vi "Subtract.vi"(7 "LabVIEW Web Service Request":refnum<class "Web Request.lvclass"> caption="LabVIEW Web服务请求", 8 "b":dbl, 11 "a":dbl) -> (2 "value":string, 3 "c":dbl)   [LabVIEW 2014]
uses:
  <vilib>/wsapi/Web Request.lvclass
panel:
  in  "variable name":string(combo) caption="变量名称"
  # "Web服务请求输入接线端用于调用“Web服务”选板的VI。除非不需要访问该选板，否则不要在连线板上删除这个输入接线端。"
  # "添加至连线板的每一个其他输入控件，在URL中对应于一个输入。如需在接线端模式输出（默认设置）下包含输出控件，则该输出控件必须与连线板相连。"
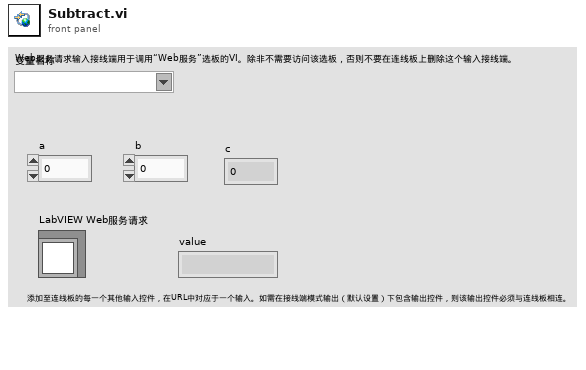
[diagram p1: front panel]
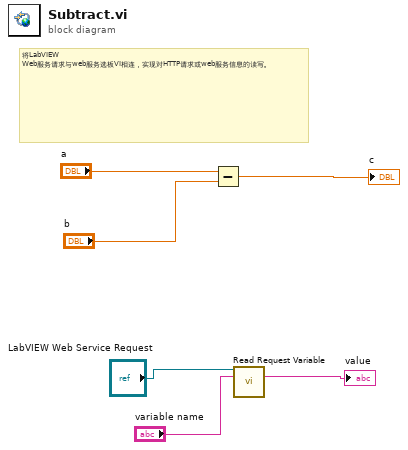
[diagram p0: block diagram]
diagram:
  # "将LabVIEW Web服务请求与web服务选板VI相连，实现对HTTP请求或web服务信息的读写。"
  n1 = Subtract(x="a", y="b") -> (x-y=→"c":dbl)
  n2 = call <vilib>:"Read Request Variable.vi"("LabVIEW Web Service Request"="LabVIEW Web Service Request", "variable name"="variable name") -> ("value"=→"value":string)  [unwired: 11 in, 2 out]
